vi "Day02-2.vi"() -> ()   [LabVIEW 2021]
panel:
  out "x*y":i32
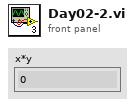
[diagram p1: front panel]
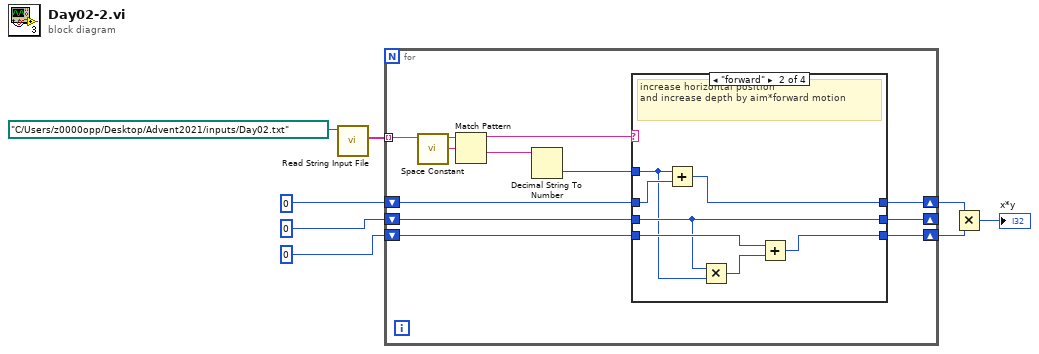
[diagram p0: block diagram]
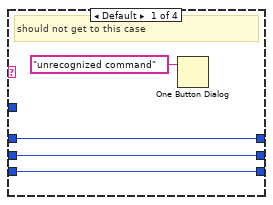
[diagram p2: hidden frame]
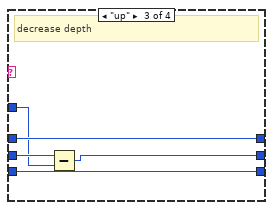
[diagram p3: hidden frame]
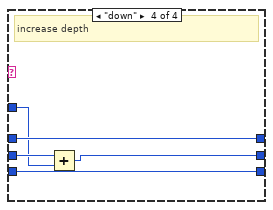
[diagram p4: hidden frame]
diagram:
  n1 = call "Read String Input File.vi"("file path (dialog if empty)"=path "C:/Users/z0000opp/Desktop/Advent2021/inputs/Day02.txt") -> ("input values"=w1:string[])  [unwired: 10 in]
  n2 = for {
    tunnel: w1 -> [w19] mode=indexing
    shift-right: [w11] -> w3
    shift-left: 0 -> [w15]
    shift-right: [w12] -> _
    shift-left: 0 -> [w14]
    shift-right: [w9] -> w4
    shift-left: 0 -> [w10]
    n3 = call <vilib>:"Space Constant.vi"() -> ("String"=w18:string)
    n4 = Match Pattern(string=w19, regular expression=w18) -> (before substring=w16:string, after substring=w17:string)  [unwired: 1 in, 2 out]
    n5 = Decimal String To Number(string=w17) -> (number=w13:i32)  [unwired: 2 in, 1 out]
    n6 = case shown="\"forward\"" w16 {
      tunnel: w15 -> [w23 w29 w35 w40]
      tunnel: w14 -> [w22 w26 w34 w39]
      tunnel: w13 -> [_ w25 w32 w37]
      tunnel: [w22 w26 w33 w38] -> w12
      tunnel: [w23 w30 w35 w40] -> w11
      tunnel: w10 -> [w20 w28 w31 w36]
      tunnel: [w20 w27 w31 w36] -> w9
      frame Default {
        # "should not get to this case"
        n7 = One Button Dialog(message="unrecognized command") -> ()  [unwired: 1 in, 1 out]
      }
      frame "forward" {
        # "increase horizontal position\nand increase depth by aim*forward motion"
        n8 = Add(x=w25, y=w29) -> (x+y=w30:i32)
        n9 = Multiply(x=w26, y=w25) -> (x*y=w24:i32)
        n10 = Add(x=w28, y=w24) -> (x+y=w27:i32)
      }
      frame "up" {
        # "decrease depth"
        n11 = Subtract(x=w34, y=w32) -> (x-y=w33:i32)
      }
      frame "down" {
        # "increase depth"
        n12 = Add(x=w39, y=w37) -> (x+y=w38:i32)
      }
    }
  }
  n13 = Multiply(x=w3, y=w4) -> (x*y=→"x*y":i32)
